vi "ArchiveResults.vi"(8 "error in":errorcluster, 10 "Archive Path":path=path "\\\\157.165.213.50\\chardata/TestResults/IdtAteResults", 11 "source path":path=path "C:/IdtATE/Results/F1150_MIXER_ATK_CORRELATION/4_19_2011/F1150_MIXER_ATK_CORRELATION_SN_6_151713.csv") -> (0 "error out":errorcluster, 2 "Filename":string="F1150_MIXER_ATK_CORRELATION_SN_6_151713.csv", 3 "Archive PathOut":path=path "\\\\157.165.213.50\\chardata/Test Results/IdtAteResults")   [LabVIEW 2018]
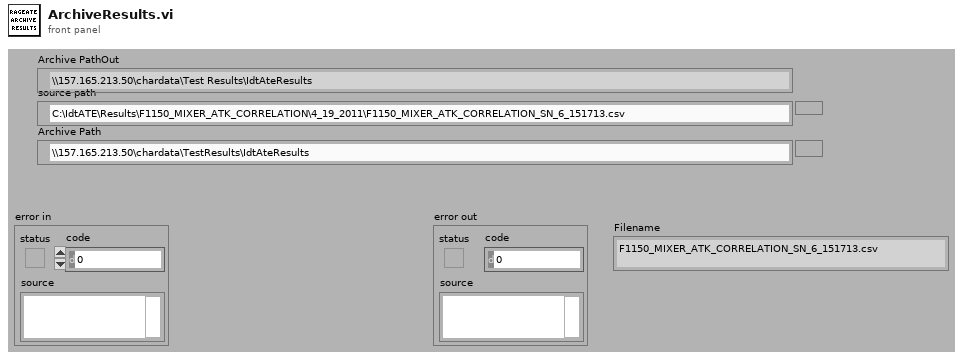
[diagram p1: front panel]
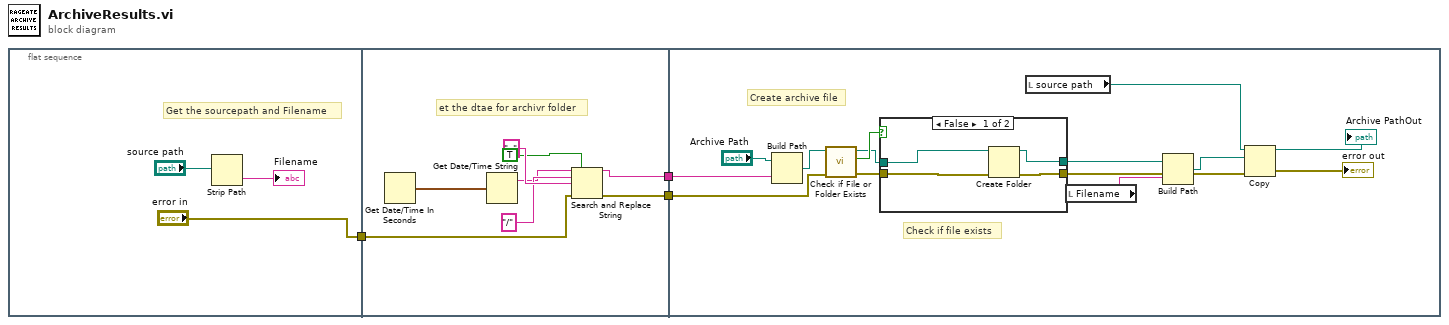
[diagram p0: block diagram]
diagram:
  n1 = flat-sequence {
    tunnel: ["error in"] -> w3
    tunnel: w3 -> [w9]
    tunnel: [w8] -> w2
    tunnel: [w7] -> w1
    tunnel: w2 -> [w27]
    tunnel: w1 -> [w18]
    frame #0 {
      # "Get the sourcepath and Filename"
      n2 = Strip Path(path="source path") -> (name=→"Filename":string)  [unwired: 1 out]
    }
    frame #1 {
      # "et the dtae for archivr folder"
      n3 = Get Date/Time In Seconds() -> (seconds since 1Jan1904=w10:timestamp)
      n4 = Get Date/Time String(seconds (now)=w10) -> (date string=w11:string)  [unwired: 2 in, 1 out]
      n5 = Search and Replace String(replace all?=TRUE ("replace all? (F)"), input string=w11, search string="/", replace string="_" ("replace string (\"\")"), error in=w9) -> (result string=w8:string, error out=w7:errorcluster)  [unwired: 3 in, 2 out]
    }
    frame #2 {
      # "Create archive file"
      # "Check if file exists"
      n6 = Build Path(base path="Archive Path", name or relative path=w27) -> (appended path=w19:path)
      n7 = call <vilib>:"Check if File or Folder Exists.vi"("error in (no error)"=w18, "path"=w19) -> ("error out"=w16:errorcluster, "file or folder exists?"=w17:bool, "dup path"=w15:path)  [unwired: 7 in]
      n8 = case shown="False" w17 {
        tunnel: w15 -> [w32 w33]
        tunnel: [w31 w33] -> w21
        tunnel: w16 -> [w30 w34]
        tunnel: [w29 w34] -> w20
        frame False {
          n9 = Create Folder(path (use dialog)=w32, error in=w30) -> (created path=w31:path, error out=w29:errorcluster)  [unwired: 1 in, 1 out]
        }
        frame True {
        }
      }
      n10 = local read "source path"() -> (w25:path)
      n11 = local read "Filename"() -> (w26:string)
      n12 = Build Path(base path=w21, name or relative path=w26) -> (appended path=w24:path)
      n13 = Copy(8:w20, 10:w24, 11:w25) -> (0:→"error out":errorcluster, 3:→"Archive PathOut":path)  [unwired: 2 in, 1 out]
    }
  }
